vi "Calc Buffer Size.vi"(8 "error in (no error)":errorcluster, 11 "Historian Module in":refnum<class "Historian Module.lvclass">) -> (0 "error out":errorcluster, 3 "Historian Module out":refnum<class "Historian Module.lvclass">)   [LabVIEW 2020, in "VolatusHistorian.lvlib" / "Historian Module.lvclass"]
uses:
  Historian Module.lvclass
  C:/dev/lv20CE/relink/lv-volatus/Volatus/Module/Module.lvclass
  VolatusConfig/Meta Type.ctl
  Historian Module.lvclass/Historian Module.ctl
  Volatus/Module/Module.lvclass/Module.ctl
  VolatusConfig/VolatusConfigElement/VolatusConfigElement.lvclass/VolatusConfigElement.ctl
  Volatus/Module/Config.vi
  VolatusConfig/VolatusConfigElement/Element.vi
  VolatusConfig/Task/Task Config.lvclass
  C:/dev/lv20CE/relink/lv-volatus/VolatusConfig/VolatusConfigElement/VolatusConfigElement.lvclass
  lv-cdm/CDM-Config/Config Lookup/Match Meta.vi
  lv-cdm/CDM-Config/Config Element/Owner.vi
  lv-cdm/CDM-Config/Config Manager/Lookup Descendant.vi
  lv-cdm/CDM-Config/Config Filter/Config Lookup.lvclass
  Volatus/Module/Module.lvclass
  VolatusConfig/VolatusConfig.lvlib
  VolatusConfig/VolatusConfigElement/VolatusConfigElement.lvclass
  lv-cdm/CDM-Config/Config Element/Config Element.lvclass
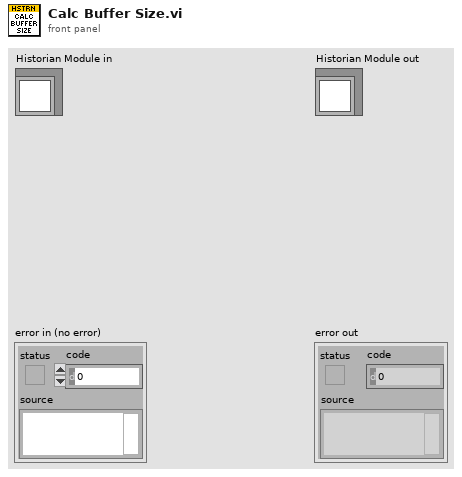
[diagram p1: front panel]
types:
  T1 = typedef "VolatusConfig.lvlib/Meta Type.ctl" = enum16{"UNKNOWN", "VL_System", "VL_Cluster", "VL_Node", "VL_Task", "VL_Group", "VL_Channel", "VL_Task_List", "VL_Scaling", "VL_Sensor", "VL_Sensor_List", "VL_Scale"}
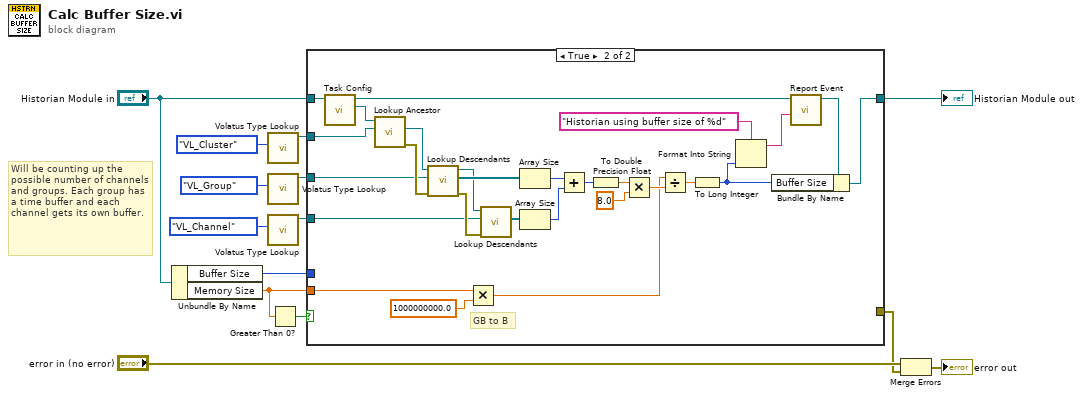
[diagram p0: block diagram]
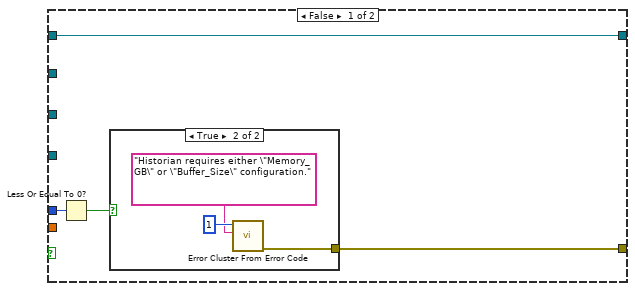
[diagram p2: hidden frame]
diagram:
  # "Will be counting up the possible number of channels and groups. Each group has a time buffer and each channel gets its own buffer."
  n1 = Unbundle By Name("Historian Module in") -> ("Buffer Size"=w11:i32, "Memory Size"=w12:dbl)
  n2 = call "Volatus Type Lookup.vi"("Meta Type"=Meta_Type."VL_Cluster") -> ("Config Lookup out"=w4:refnum<class "Config Lookup.lvclass">)  [unwired: 9 in, 1 out]
  n3 = call "Volatus Type Lookup.vi"("Meta Type"=Meta_Type."VL_Group") -> ("Config Lookup out"=w5:refnum<class "Config Lookup.lvclass">)  [unwired: 9 in, 1 out]
  n4 = call "Volatus Type Lookup.vi"("Meta Type"=Meta_Type."VL_Channel") -> ("Config Lookup out"=w6:refnum<class "Config Lookup.lvclass">)  [unwired: 9 in, 1 out]
  n5 = Greater Than 0?(x=w12) -> (x > 0?=w13:bool)
  n6 = case shown="True" w13 {
    tunnel: w12 -> [_ w32]
    tunnel: w11 -> [w18 _]
    tunnel: "Historian Module in" -> [w16 w46]
    tunnel: w6 -> [_ w39]
    tunnel: w5 -> [_ w38]
    tunnel: w4 -> [_ w37]
    tunnel: [w16 w29] -> w3
    tunnel: [w15 _] -> w1
    frame False {
      n7 = Less Or Equal To 0?(x=w18) -> (x <= 0?=w17:bool)
      n8 = case shown="True" w17 {
        tunnel: [_ w19] -> w15
        frame False {
        }
        frame True {
          n9 = call <vilib>:"Error Cluster From Error Code.vi"("error message (\"\")"="Historian requires either \"Memory_GB\" or \"Buffer_Size\" configuration.", "error code (0)"=1) -> ("error out"=w19:errorcluster)  [unwired: 7 in]
        }
      }
    }
    frame True {
      # "GB to B"
      n10 = call "Task Config.vi"("Module in"=w46) -> ("Task Config"=w45:refnum<class "Task Config.lvclass">, "Module out"=w30:refnum<class "Historian Module.lvclass">)  [unwired: 8 in, 1 out]
      n11 = call "Lookup Ancestor.vi"("Lookup"=w37, "VolatusConfigElement in"=w45) -> ("error out"=w47:errorcluster, "Ancestor"=w44:refnum<class "Config Element.lvclass">)  [unwired: 7 in, 1 out]
      n12 = call "Lookup Descendants.vi"("error in (no error)"=w47, "Lookup"=w38, "Config Element in"=w44) -> ("error out"=w48:errorcluster, "Descendants"=w42:refnum<class "Config Element.lvclass">[], "Config Element out"=w24:refnum<class "Config Element.lvclass">)  [unwired: 6 in]
      n13 = Multiply(x=w32, y=1000000000.0) -> (x*y=w23:dbl)
      n14 = call "Lookup Descendants.vi"("error in (no error)"=w48, "Lookup"=w39, "Config Element in"=w24) -> ("Descendants"=w43:refnum<class "Config Element.lvclass">[])  [unwired: 6 in, 2 out]
      n15 = Array Size(array=w42) -> (size(s)=w41:i32)
      n16 = Array Size(array=w43) -> (size(s)=w40:i32)
      n17 = Add(x=w41, y=w40) -> (x+y=w36:i32)
      n18 = To Double Precision Float(number=w36) -> (double precision float=w35:dbl)
      n19 = Multiply(x=w35, y=8.0) -> (x*y=w33:dbl)
      n20 = Divide(x=w23, y=w33) -> (x/y=w31:dbl)
      n21 = To Long Integer(number=w31) -> (32bit integer=w27:i32)
      n22 = Format Into String(format string="Historian using buffer size of %d", w27) -> (resulting string=w25:string)  [unwired: 2 in, 1 out]
      n23 = call "Report Event.vi"("Message"=w25, "Module in"=w30) -> ("Module out"=w26:refnum<class "Historian Module.lvclass">)  [unwired: 8 in, 1 out]
      n24 = Bundle By Name(cluster=w26, "Buffer Size"=w27) -> (w29:refnum<class "Historian Module.lvclass">)
    }
  }
  "Historian Module out" <- w3
  n25 = Merge Errors("error in (no error)", w1) -> (→"error out":errorcluster)
